vi "Prepare_Scan_Routine_Aging.vi"(0 "JV curve scan settings In":T1(array[cluster]), 1 "Cell to be measured In":T2) -> (2 "VISA resource name out":refnum<visa-resource-name>, 3 "error out":errorcluster, 4 "JV curve scan settings Out":T1(array[cluster]), 5 "Cell to be measured Out":T2)   [LabVIEW 2011]
uses:
  Sweep Routine v5.0 Folder/Y/DAQ/Condensed Matter/HJSGroup/LabView/Solar Simulator/Archive/Solar Sim v4.0/Instrument Drivers/Keithley 24XX/Public/Data/Read (Single Point).vi
  Sweep Routine v5.0 Folder/Y/DAQ/Condensed Matter/HJSGroup/LabView/Solar Simulator/Archive/Solar Sim v4.0/Instrument Drivers/Keithley 24XX/Keithley 24XX.lvlib
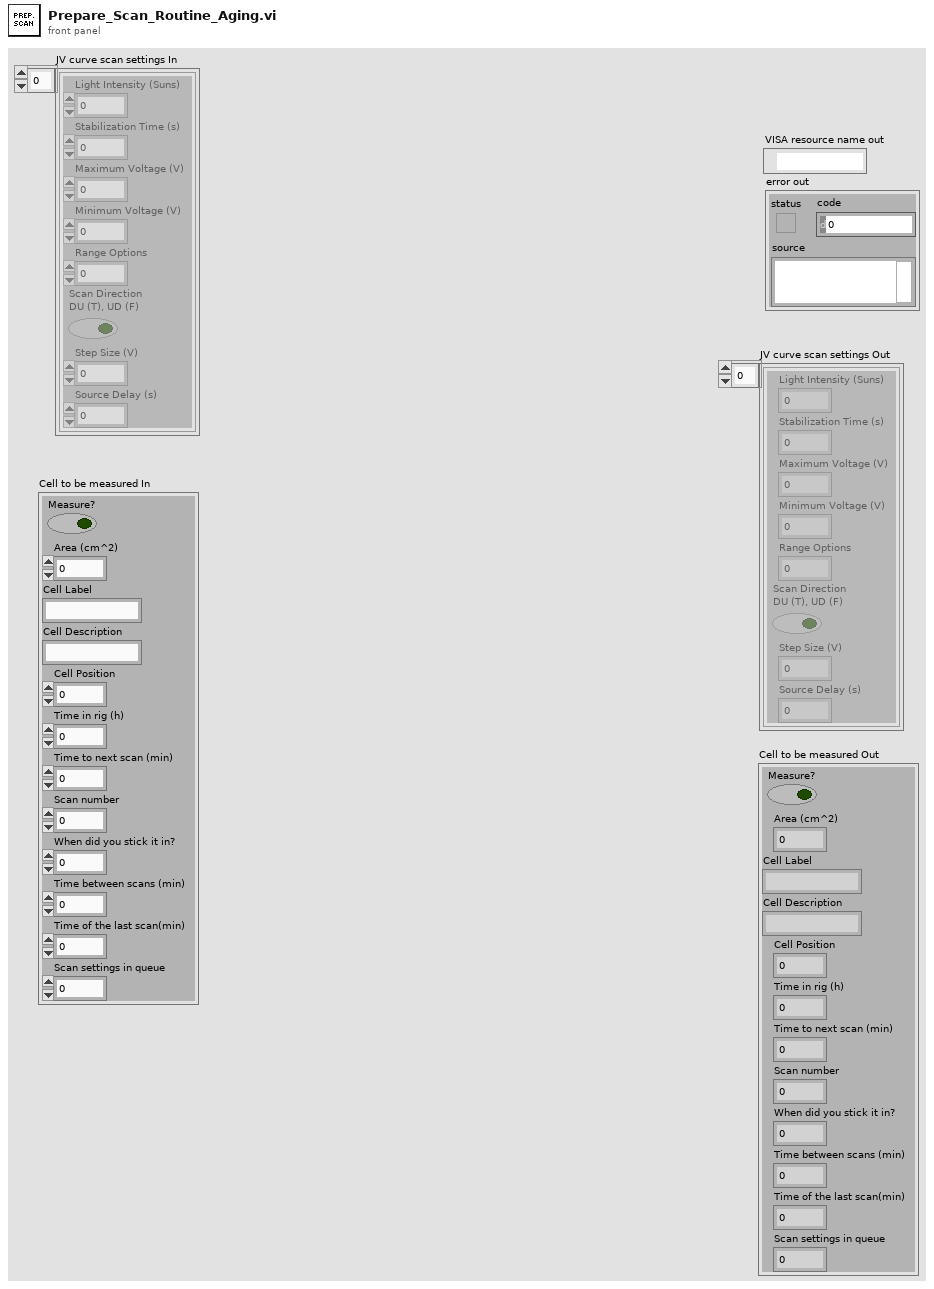
[diagram p1: front panel]
types:
  T1 = cluster{"Light Intensity (Suns)":dbl, "Stabilization Time (s)":dbl, "Maximum Voltage (V)":dbl, "Minimum Voltage (V)":dbl, "Range Options":u16, "Scan Direction\nDU (T), UD (F)":bool, "Step Size (V)":dbl, "Source Delay (s)":dbl}[]
  T2 = cluster{"Measure?":bool, "Area (cm^2)":dbl, "Cell Label":string, "Cell Description":string, "Cell Position":i32, "Time in rig (h)":dbl, "Time to next scan (min)":dbl, "Scan number":dbl, "When did you stick it in?":dbl, "Time between scans (min)":dbl, "Time of the last scan(min)":dbl, "Scan settings in queue":u16}
  T3 = cluster{"Baud Rate":u32, "Parity":u16, "Data Bits":u16, "Stop Bits":u16, "Flow Control":u16}
  T4 = cluster{"Light Intensity (Suns)":dbl, "Stabilization Time (s)":dbl, "Maximum Voltage (V)":dbl, "Minimum Voltage (V)":dbl, "Range Options":u16, "Scan Direction\nDU (T), UD (F)":bool, "Step Size (V)":dbl, "Source Delay (s)":dbl}
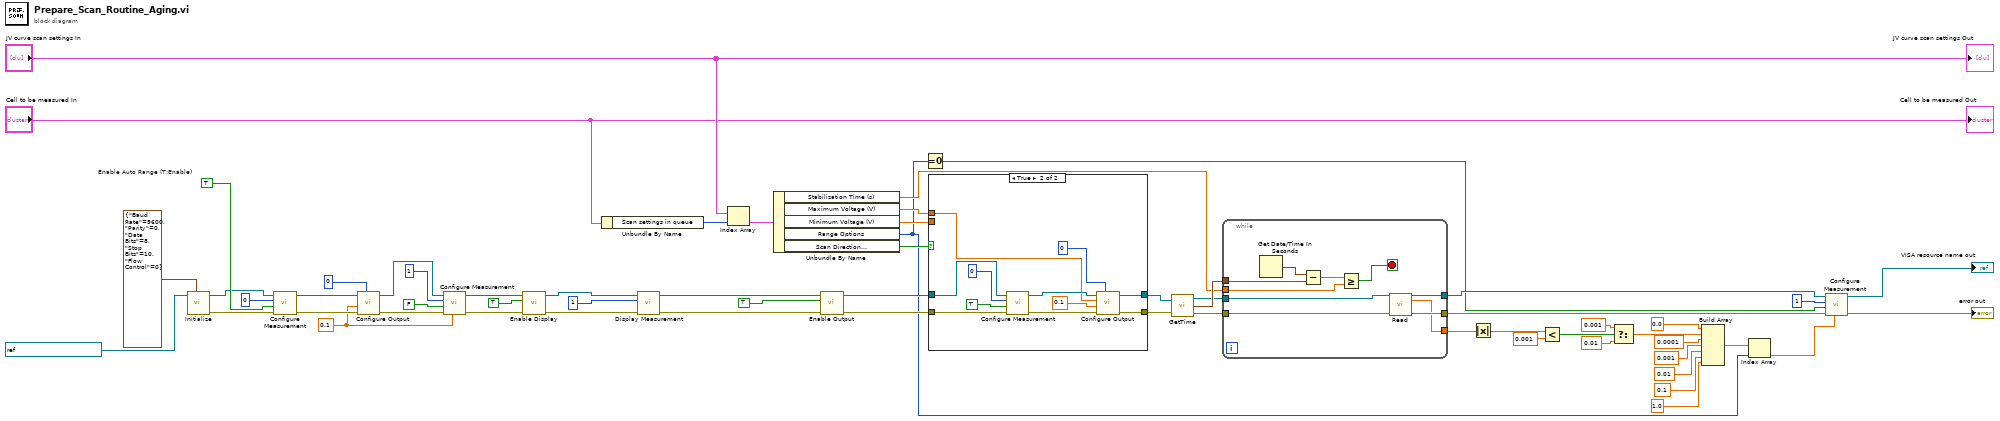
[diagram p0: block diagram]
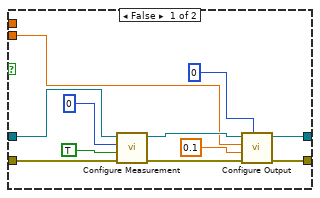
[diagram p2: hidden frame]
diagram:
  w29 = 0.1 ("Compliance  Level (0.1)")
  w50 = TRUE  # Enable Auto Range (T:Enable)
  n1 = call "Initialize.vi"("Serial Configuration"=T3 {"Baud Rate"=9600, "Parity"=0, "Data Bits"=8, "Stop Bits"=10, "Flow Control"=0}, "VISA resource name"=refnum<visa-resource-name> "KE2400ExampleInstr") -> ("error out"=w45:errorcluster, "VISA resource name out"=w44:refnum<visa-resource-name>)  [unwired: 3 in, 5 out]
  n2 = call "Configure Measurement.vi"("error in (no error)"=w45, "Enable Auto Range (T:Enable)"=w50, "Function (0: Volts)"=0, "VISA resource name"=w44) -> ("error out"=w46:errorcluster, "VISA resource name out"=w49:refnum<visa-resource-name>)  [unwired: 1 in, 5 out]
  n3 = call "Configure Output.vi"("Source Mode  (0: Voltage)"=0, "error in (no error)"=w46, "Compliance  Level (0.1)"=w29, "VISA resource name"=w49) -> ("error out"=w47:errorcluster, "VISA resource name out"=w48:refnum<visa-resource-name>)  [unwired: 2 in, 4 out]
  n4 = call "Configure Measurement.vi"("Manual Range (1.0)"=w29, "error in (no error)"=w47, "Enable Auto Range (T:Enable)"=FALSE, "Function (0: Volts)"=1, "VISA resource name"=w48) -> ("error out"=w42:errorcluster, "VISA resource name out"=w43:refnum<visa-resource-name>)  [unwired: 5 out]
  n5 = call "Enable Display.vi"("error in (no error)"=w42, "Enable Display (T: Enable)"=TRUE ("Enable Output (T: Enable)"), "VISA resource name"=w43) -> ("error out"=w54:errorcluster, "VISA resource name out"=w55:refnum<visa-resource-name>)  [unwired: 7 out]
  n6 = Unbundle By Name("Cell to be measured In") -> ("Scan settings in queue"=w9:u16)
  n7 = call "Display Measurement.vi"("error in (no error)"=w54, "Displayed Measurement (0: Voltage)"=1, "VISA resource name"=w55) -> ("error out"=w53:errorcluster, "VISA resource name out"=w56:refnum<visa-resource-name>)  [unwired: 7 out]
  n8 = Index Array(array="JV curve scan settings In", index=w9) -> (element=w8:T4)
  n9 = Unbundle By Name(w8) -> ("Stabilization Time (s)"=w4:dbl, "Maximum Voltage (V)"=w7:dbl, "Minimum Voltage (V)"=w6:dbl, "Range Options"=w3:u16, "Scan Direction\nDU (T), UD (F)"=w5:bool)
  n10 = call "Enable Output.vi"("error in (no error)"=w53, "Enable Output (T: Enable)"=TRUE, "VISA resource name"=w56) -> ("error out"=w39:errorcluster, "VISA resource name out"=w40:refnum<visa-resource-name>)  [unwired: 7 out]
  n11 = Equal To 0?(x=w3) -> (x = 0?=w20:bool)
  n12 = case shown="True" w5 {
    tunnel: w40 -> [w66 w78]
    tunnel: [w68 w76] -> w36
    tunnel: [w67 w75] -> w37
    tunnel: w39 -> [w65 w77]
    tunnel: w7 -> [_ w73]
    tunnel: w6 -> [w63 _]
    frame False {
      n13 = call "Configure Measurement.vi"("error in (no error)"=w65, "Enable Auto Range (T:Enable)"=TRUE, "Function (0: Volts)"=0, "VISA resource name"=w66) -> ("error out"=w70:errorcluster, "VISA resource name out"=w71:refnum<visa-resource-name>)  [unwired: 1 in, 5 out]
      n14 = call "Configure Output.vi"("Source Mode  (0: Voltage)"=0, "error in (no error)"=w70, "Compliance  Level (0.1)"=0.1, "Output Level (0)"=w63, "VISA resource name"=w71) -> ("error out"=w67:errorcluster, "VISA resource name out"=w68:refnum<visa-resource-name>)  [unwired: 1 in, 4 out]
    }
    frame True {
      n15 = call "Configure Measurement.vi"("error in (no error)"=w77, "Enable Auto Range (T:Enable)"=TRUE, "Function (0: Volts)"=0, "VISA resource name"=w78) -> ("error out"=w81:errorcluster, "VISA resource name out"=w82:refnum<visa-resource-name>)  [unwired: 1 in, 5 out]
      n16 = call "Configure Output.vi"("Source Mode  (0: Voltage)"=0, "error in (no error)"=w81, "Compliance  Level (0.1)"=0.1, "Output Level (0)"=w73, "VISA resource name"=w82) -> ("error out"=w75:errorcluster, "VISA resource name out"=w76:refnum<visa-resource-name>)  [unwired: 1 in, 4 out]
    }
  }
  n17 = call "GetTime.vi"("VISA resource name"=w36, "error in"=w37) -> ("VISA resource name out"=w34:refnum<visa-resource-name>, "current time"=w38:timestamp, "error out"=w35:errorcluster)
  n18 = while {
    tunnel: w34 -> [w92]
    tunnel: [w91] -> w27
    tunnel: w35 -> [w90]
    tunnel: [w89] -> w26
    tunnel: w4 -> [w88]
    tunnel: w38 -> [w85]
    tunnel: [w83] -> w22
    stop <- w87 stop-if-true
    n19 = Get Date/Time In Seconds() -> (seconds since 1Jan1904=w86:timestamp)
    n20 = Subtract(x=w86, y=w85) -> (x-y=w84:dbl)
    n21 = Greater Or Equal?(x=w84, y=w88) -> (x >= y?=w87:bool)
    n22 = call-poly "Read.vi"("VISA resource name"=w92, "error in (no error)"=w90) -> ("VISA resource name out"=w91:refnum<visa-resource-name>, "Current"=w83:sgl, "error out"=w89:errorcluster)  [unwired: 2 in, 9 out]
  }
  n23 = Absolute Value(x=w22) -> (abs(x)=w21:sgl)
  n24 = Less?(x=w21, y=0.001) -> (x < y?=w32:bool)
  n25 = Select(t=0.001, s=w32, f=0.01) -> (s? t:f=w19:dbl)
  n26 = Build Array(0.0 ("s? t:f"), w19, 0.0001 ("s? t:f"), 0.001 ("s? t:f"), 0.01 ("s? t:f"), 0.1 ("s? t:f"), 1.0 ("s? t:f")) -> (w12:dbl[])
  n27 = Index Array(array=w12, index=w3) -> (element=w11:dbl)
  n28 = call "Configure Measurement.vi"("Manual Range (1.0)"=w11, "error in (no error)"=w26, "Enable Auto Range (T:Enable)"=w20, "Function (0: Volts)"=1, "VISA resource name"=w27) -> ("error out"=→"error out":errorcluster, "VISA resource name out"=→"VISA resource name out":refnum<visa-resource-name>)  [unwired: 5 out]
  "Cell to be measured Out" <- "Cell to be measured In"
  "JV curve scan settings Out" <- "JV curve scan settings In"
